vi "Configure RF Upconversion.vi"(7 "User Defined Frequency (28GHz)":dbl=28000000000.0 format="%#.9p", 8 "error in (no error)":errorcluster, 9 "Phase Compensation (Off)":i32(ring) items=["Off", "Carrier Freq", "User Defined"], 10 "Instance (1)":T1=1, 11 "VISA resource name":refnum<visa-resource-name>) -> (0 "error out":errorcluster, 3 "VISA resource name out":refnum<visa-resource-name>)   [LabVIEW 2015, in "Rohde&Schwarz CMXP NR FR2 Measurement.lvlib"]
doc: "Specifies the phase compensation applied by the UE during the modulation and upconversion.\n\nAttribute:\nRSCMXPNRFR2M_ATTR_RF_UPCONVERSION\n\nRemote-control command:\nCONFigure:NRMMw:MEAS<i>:MEValuation:PCOMp"
uses:
  <instrlib>/Rohde&Schwarz CMXP NR FR2 Measurement/Rohde&Schwarz CMXP NR FR2 Measurement.lvlib
  <instrlib>/Rohde&Schwarz CMXP NR FR2 Measurement/Private/_Instance.ctl
  <instrlib>/Rohde&Schwarz CMXP NR FR2 Measurement/Private/rsidr_core.llb/rsidr_core.lvlib
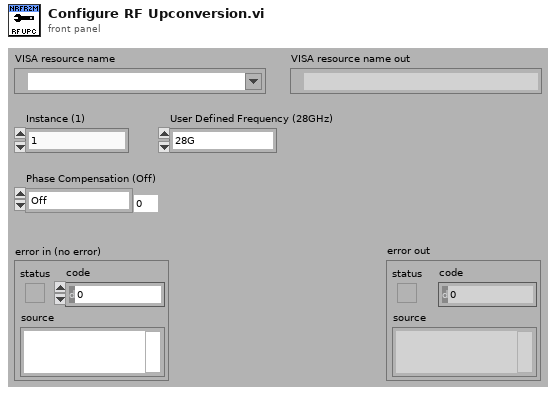
[diagram p1: front panel]
types:
  T1 = typedef "Rohde&Schwarz CMXP NR FR2 Measurement.lvlib/_Instance.ctl" = i32
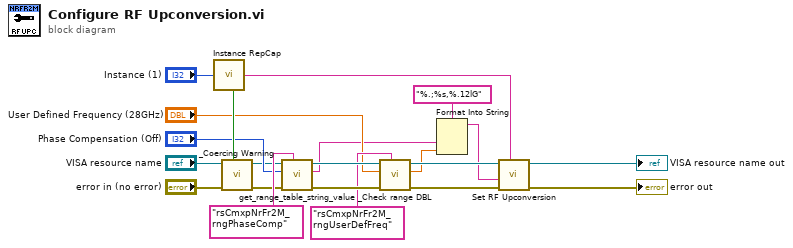
[diagram p0: block diagram]
diagram:
  n1 = call <instrlib>:"Instance RepCap.vi"("Instance In"="Instance (1)") -> ("In Range?"=w19:bool, "RepCap Identifier Out"=w7:string)  [unwired: 1 in]
  n2 = call <instrlib>:"_Coercing Warning.vi"("In Range?"=w19, "error in (no error)"="error in (no error)", "VISA resource name"="VISA resource name") -> ("error out"=w15:errorcluster, "VISA resource name out"=w16:refnum<visa-resource-name>)  [unwired: 7 in]
  n3 = call <instrlib>:"get_range_table_string_value.vi"("Range Table ID in"="rsCmxpNrFr2M_rngPhaseComp", "error in"=w15, "I32 input"="Phase Compensation (Off)", "VISA resource name"=w16) -> ("error out"=w14:errorcluster, "String Value out"=w4:string, "VISA resource name out"=w13:refnum<visa-resource-name>)  [unwired: 5 in]
  n4 = call <instrlib>:"_Check range DBL.vi"("Range Table Identifier"="rsCmxpNrFr2M_rngUserDefFreq", "error in (no error)"=w14, "DBL Value In"="User Defined Frequency (28GHz)", "VISA resource name"=w13) -> ("error out"=w10:errorcluster, "DBL Value Out"=w3:dbl, "VISA resource name out"=w9:refnum<visa-resource-name>)  [unwired: 5 in]
  n5 = Format Into String(format string="%.;%s,%.12lG", w4, w3) -> (resulting string=w1:string)  [unwired: 2 in, 1 out]
  n6 = call "Set RF Upconversion"("Repeated Capabilities"=w7, "error in (no error)"=w10, "RF Upconversion ()"=w1, "instrument handle"=w9) -> ("error out"=→"error out":errorcluster, "instrument handle out"=→"VISA resource name out":refnum<visa-resource-name>)  [unwired: 6 in]
